vi "Write Element of Cameras.vi"(8 "error in (no error)":errorcluster, 9 "Camera":cluster{"Name":string, "IMAQ Session":T1}, 10 "index":i32, 11 "Gantry Class in":refnum<class "Gantry Class.lvclass">) -> (0 "error out":errorcluster, 3 "Gantry Class out":refnum<class "Gantry Class.lvclass">)   [LabVIEW 2011, in "Gantry Class.lvclass"]
uses:
  Gantry Class.lvclass
  <vilib>/userdefined/High Color/IMAQdx.ctl
  Gantry Class.lvclass/Gantry Class.ctl
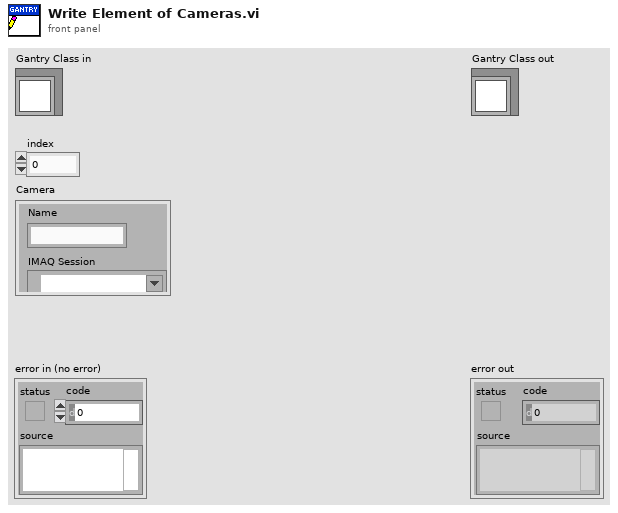
[diagram p1: front panel]
types:
  T1 = typedef "IMAQdx.ctl" = refnum<k21>
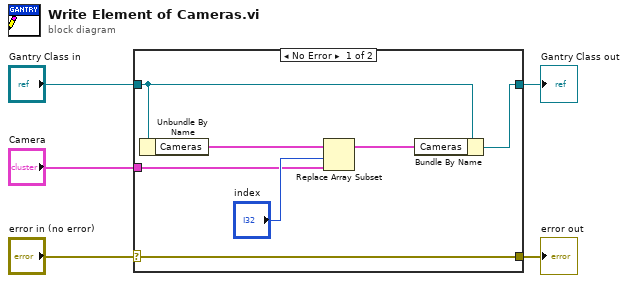
[diagram p0: block diagram]
diagram:
  n1 = case shown="No Error" "error in (no error)" {
    selector: "error in (no error)" -> [w12 w13]
    tunnel: [w12 w13] -> w4
    tunnel: [w11 w14] -> w2
    tunnel: "Gantry Class in" -> [w10 w14]
    tunnel: "Camera" -> [w6 _]
    frame No Error {
      n2 = Unbundle By Name(w10) -> ("Cameras"=w9:cluster{"Name":string, "IMAQ Session":T1}[])
      n3 = Replace Array Subset(array=w9, new element=w6, index="index") -> (w8:cluster{"Name":string, "IMAQ Session":T1}[])
      n4 = Bundle By Name(cluster=w10, "Cameras"=w8) -> (w11:refnum<class "Gantry Class.lvclass">)
    }
    frame Error {
    }
  }
  "error out" <- w4
  "Gantry Class out" <- w2
